vi "全局 1.vi"() -> ()   [LabVIEW 2016]
panel:
  in  "机种":string
  in  "KukaIP":string
  out "Exit":bool
  out "Pause":bool
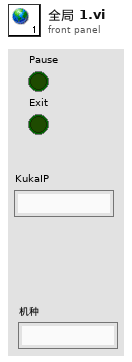
[diagram p1: front panel]
diagram:
